vi "FPGA Main.vi"() -> ()   [LabVIEW 2019]
doc: "Main FPGA VI\nUse the bitfile generated by this VI in the real-time code.\n\nFlip the channels for input and output"
uses:
  TypeDefs/SamplingModeEnum.ctl
  <vilib>/rvi/Emulation/niFpgaGetClockAttributes.vi
  <vilib>/rvi/Emulation/niFpgaSctlEmulationGetInTimedLoop.vi
  <vilib>/rvi/Emulation/niFpgaEmulationReportErrorSimple.vi
  <vilib>/rvi/Emulation/niFpgaEmulationIsFPGAContextNoSignature.vi
  <vilib>/rvi/errors/niFpgaSetErrorForExecOnDevCompSimple.vi
  <vilib>/rvi/eio/common/nirviEmuReportErrorAndStop.vi
  <vilib>/rvi/DataTransferAndStorage/Container/Common/niFpgaContainerGetUniqueNameForEmu.vi
  <vilib>/rvi/FIFO/Fifo_Resource/nirvififoEmulationSetSize.vi
  <vilib>/rvi/FIFO/Fifo_Resource/nirviFifoEmulationQueueMgr.vi
  <instcachedir>/0/nirviFifoEmulationQueueMgr_E5CAEC123FF24DC58D834DCA3CDAA9B5.lvgen/nirviFifoEmulationQueueMgr_E5CAEC123FF24DC58D834DCA3CDAA9B5_003.vi
  <vilib>/rvi/FIFO/Fifo_Resource/nirvififoEmulationDetermineInputValidOut.vi
  <vilib>/rvi/FIFO/Fifo_Resource/nirvififoEmulationCreateLock.vi
  <vilib>/rvi/Emulation/niFpgaProcessEmulError.vi
  <vilib>/rvi/FIFO/Fifo_Resource/nirvififoEmulationObtainLock.vi
  <vilib>/rvi/FIFO/Fifo_Resource/nirvififoEmulationReleaseLock.vi
  <vilib>/rvi/occurrence/nirviWaitOnOccurrenceBase.vi
  <vilib>/rvi/errors/nirviReportUnexpectedCaseInternalError.vi
  <vilib>/rvi/errors/nirviReportUnexpectedCaseInternalError (U32).vi
  <vilib>/rvi/eio/common/nirviEmuTemplateMethod_errors.vi
  <vilib>/rvi/Emulation/niFpgaCriticalErrorInLSC.vi
  <vilib>/Utility/error.llb/Clear Errors.vi
  <vilib>/rvi/DataTransferAndStorage/Container/XNode/niFpgaContainer.xnode
  <vilib>/rvi/FIFO/Fifo_Resource/nirvififoEmulationWrite.vi
  <vilib>/eio/EIONode/EIONode.xnode
  <vilib>/rvi/Analysis/measure/butterworth/XNode/niFpgaButterworthFilter.xnode
  <vilib>/rvi/FIFO/Fifo_Resource/nirvififoEmulationRead.vi
  FPGA functions/FPGA functions.lvlib
panel:
  in  "Sampling Mode":T1
  out "Int. Output":i16
  out "Raw Int. Input":i16
  in  "Bit-resolution":i8=12
  in  "Sample Time [us]":u32=3
  out "AO Loop time [us]":u32
  in  "AO Out [V]":fxp<+/-,18,5> format="%#.6g"
  in  "AO enable?":bool
  out "AI In [V]":fxp<+/-,18,5> format="%#.6g"
  out "AI Loop time [us]":u32
  out "FPGA AO DMA\nOverflow?":bool
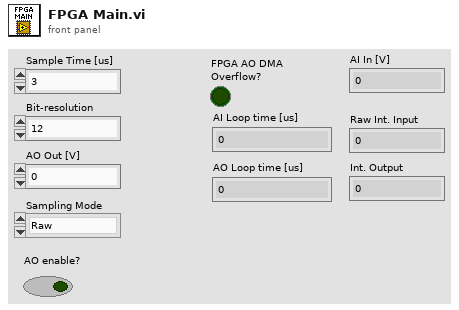
[diagram p1: front panel]
types:
  T1 = typedef "SamplingModeEnum.ctl" = enum16{"Raw", "LPF", "4 pt. Avg. + LPF"}
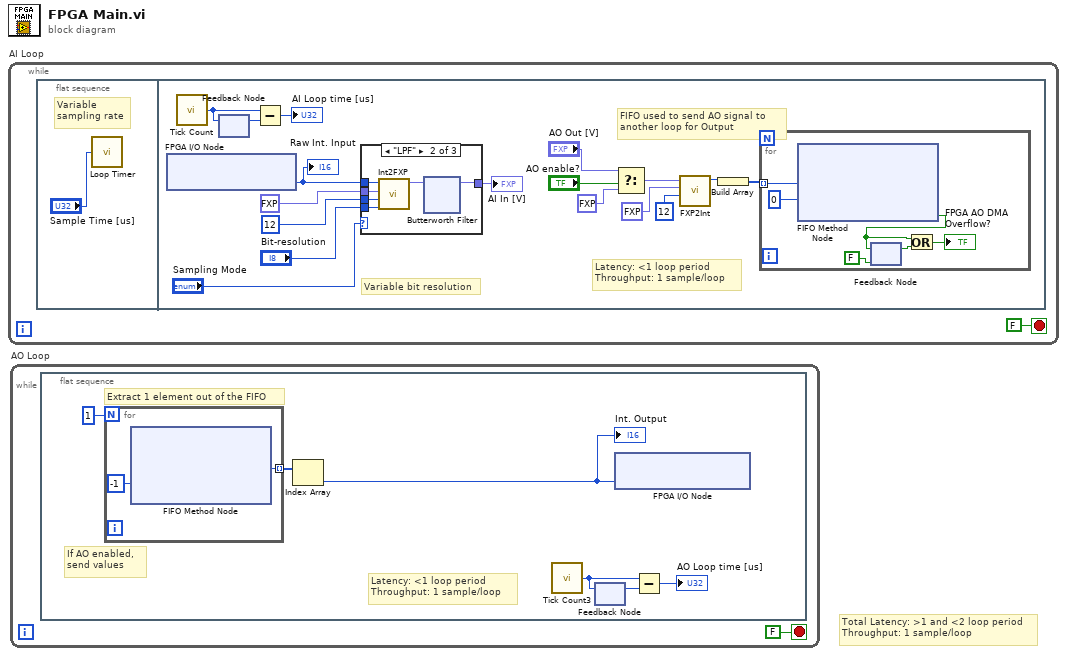
[diagram p0: block diagram]
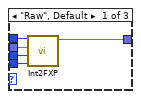
[diagram p2: hidden frame]
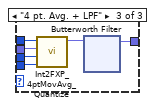
[diagram p3: hidden frame]
diagram:
  # "Total Latency: >1 and <2 loop period\nThroughput: 1 sample/loop"
  n1 = while "AI Loop" {
    stop <- FALSE stop-if-true
    n2 = flat-sequence {
      frame #0 {
        # "Variable\nsampling rate"
        n3 = call "Loop Timer"("Count(uSec)"="Sample Time [us]") -> ()  [unwired: 1 out]
      }
      frame #1 {
        # "Variable bit resolution"
        # "Latency: <1 loop period\nThroughput: 1 sample/loop"
        # "FIFO used to send AO signal to \nanother loop for Output"
        n4 = xnode "FPGA I/O Node"() -> ("ConnectorC/AI0"=w4:i16)  [unwired: 1 in, 1 out]
        "Raw Int. Input" <- w4
        n5 = call "Tick Count"() -> ("Tick Count(uSec)"=w19:u32)
        n6 = feedback #1() -> (w18:u32)  [unwired: 1 in]
        n7 = feedback-in #1(w19) -> ()
        n8 = Subtract(x=w19, y=w18) -> (x-y=→"AI Loop time [us]":u32)
        n9 = case shown="\"LPF\"" "Sampling Mode" {
          tunnel: [w24 w25 w39] -> w16
          tunnel: i8 12 ("Input Bit resolution") -> [w23 w28 w42]
          tunnel: fxp<+,8,4> 10.0 ("Multiplier") -> [w22 w29 w43]
          tunnel: "Bit-resolution" -> [w21 w27 w41]
          tunnel: w4 -> [w20 w30 w38]
          frame "Raw", Default {
            n10 = call "Int2FXP.vi"("Output Bit resolution"=w21, "Input Bit resolution"=w23, "Multiplier"=w22, "Input (Int)"=w20) -> ("Output (FXP)"=w24:fxp<+/-,18,5>)  [unwired: 7 in]
          }
          frame "LPF" {
            n11 = call "Int2FXP.vi"("Output Bit resolution"=w27, "Input Bit resolution"=w28, "Multiplier"=w29, "Input (Int)"=w30) -> ("Output (FXP)"=w26:fxp<+/-,18,5>)  [unwired: 7 in]
            n12 = xnode "Butterworth Filter"("input data"=w26) -> ("output data"=w25:fxp<+/-,18,5>)  [unwired: 2 in]
          }
          frame "4 pt. Avg. + LPF" {
            n13 = call "Int2FXP_4ptMovAvg_Quantize.vi"("Output Bit resolution"=w41, "Input Bit resolution"=w42, "Multiplier"=w43, "Input (Int)"=w38) -> ("Output (FXP)"=w40:fxp<+/-,18,5>)  [unwired: 7 in]
            n14 = xnode "Butterworth Filter"("input data"=w40) -> ("output data"=w39:fxp<+/-,18,5>)  [unwired: 2 in]
          }
        }
        "AI In [V]" <- w16
        n15 = Select(t="AO Out [V]", s="AO enable?", f=fxp<+/-,18,5> 0.0) -> (s? t:f=w6:fxp<+/-,18,5>)
        n16 = call "FXP2Int.vi"("Output Bit resolution"=i8 12 ("Bit resolution"), "Multiplier"=fxp<+,18,-1> 0.10000038146972656, "Input (FXP)"=w6) -> ("Output (Int)"=w15:i16)  [unwired: 8 in]
        n17 = Build Array(w15) -> (w8:i16[])
        n18 = for {
          tunnel: w8 -> [w53] mode=indexing
          n19 = xnode ("FIFO Method Node")("Element"=w53, "Timeout"=0) -> ("Timed Out?"=w51:bool)  [unwired: 1 in, 1 out]
          n20 = feedback-in #2(w51) -> ()
          n21 = feedback #2(FALSE ("Timed Out?")) -> (w55:bool)
          n22 = Or(x=w51, y=w55) -> (x .or. y?=→"FPGA AO DMA\nOverflow?":bool)
        }
      }
    }
  }
  n23 = while "AO Loop" {
    stop <- FALSE stop-if-true
    n24 = flat-sequence {
      frame #0 {
        # "Latency: <1 loop period\nThroughput: 1 sample/loop"
        # "If AO enabled, \nsend values"
        # "Extract 1 element out of the FIFO"
        n25 = for {
          N: 1 -> [_]
          tunnel: [w65] -> w60 mode=indexing
          n26 = xnode ("FIFO Method Node")("Timeout"=-1) -> ("Element"=w65:i16)  [unwired: 1 in, 2 out]
        }
        n27 = Index Array(array=w60) -> (element=w58:i16)  [unwired: 1 in]
        "Int. Output" <- w58
        n28 = call "Tick Count3"() -> ("Tick Count(uSec)"=w63:u32)
        n29 = feedback #3() -> (w62:u32)  [unwired: 1 in]
        n30 = feedback-in #3(w63) -> ()
        n31 = xnode "FPGA I/O Node"("ConnectorC/AO0"=w58) -> ()  [unwired: 1 in, 1 out]
        n32 = Subtract(x=w63, y=w62) -> (x-y=→"AO Loop time [us]":u32)
      }
    }
  }
